vi "Read.vi"(10 "Address":u16 format="%.0x", 11 "EEPROM in":refnum<class "RAM.lvclass">) -> (3 "Data":u8 format="%02x")   [LabVIEW 2021, in "RAM.lvclass"]
uses:
  RAM.lvclass
  RAM.lvclass/RAM.ctl
panel:
  out "x .and. y?":u16
  out "EEPROM":u8[](array[numeric]) format="%.0x"
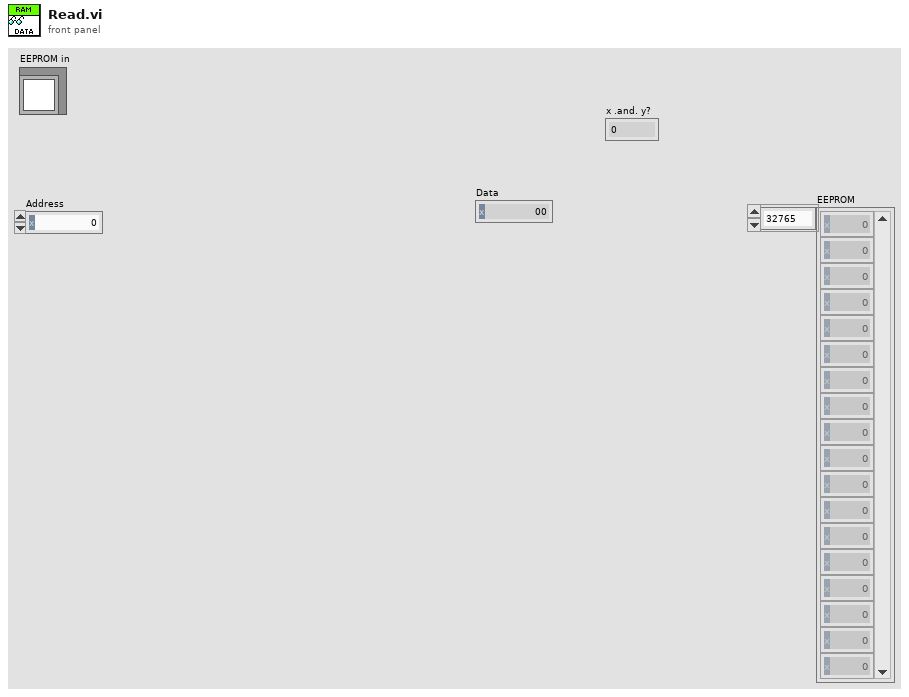
[diagram p1: front panel]
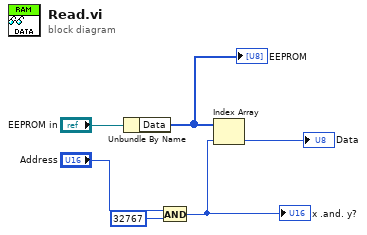
[diagram p0: block diagram]
diagram:
  n1 = Unbundle By Name("EEPROM in") -> ("Data"=w4:u8[])
  "EEPROM" <- w4
  n2 = And(x="Address", y=u16 32767) -> (x .and. y?=w1:u16)
  "x .and. y?" <- w1
  n3 = Index Array(array=w4, index=w1) -> (element=→"Data":u8)
